vi "OverwriteIni.vi"() -> ()   [LabVIEW 2019]
uses:
  <vilib>/Utility/config.llb/NI_LVConfig.lvlib
  <vilib>/Utility/config.llb/Read Key (String).vi
panel:
  in  "configuration file path":path
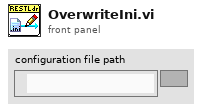
[diagram p1: front panel]
types:
  T1 = typedef "NI_LVConfig.lvlib/Config Data RefNum.ctl" = refnum<k1>
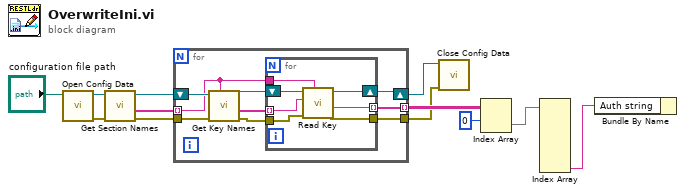
[diagram p0: block diagram]
diagram:
  n1 = call <vilib>:"Open Config Data.vi"("configuration file path"="configuration file path") -> ("error out"=w10:errorcluster, "refnum"=w11:T1)  [unwired: 8 in, 1 out]
  n2 = call <vilib>:"Get Section Names.vi"("error in (no error)"=w10, "refnum"=w11) -> ("error out"=w9:errorcluster, "section names"=w7:string[], "refnum out"=w8:T1)  [unwired: 7 in]
  n3 = for {
    tunnel: w7 -> [w16] mode=indexing
    shift-right: [w18] -> w5
    shift-left: w8 -> [w20]
    tunnel: w9 -> [w21]
    tunnel: [w15] -> w4
    tunnel: [w13] -> w6 mode=indexing
    n4 = call <vilib>:"Get Key Names.vi"("section"=w16, "error in (no error)"=w21, "refnum"=w20) -> ("error out"=w14:errorcluster, "key names"=w17:string[], "refnum out"=w19:T1)  [unwired: 5 in, 1 out]
    n5 = for {
      shift-right: [w27] -> w18
      shift-left: w19 -> [w28]
      tunnel: w17 -> [w26] mode=indexing
      tunnel: w16 -> [w25]
      tunnel: [w24] -> w15
      tunnel: w14 -> [w23]
      tunnel: [w22] -> w13 mode=indexing
      n6 = call-poly <vilib>:"Read Key.vi"("section"=w25, "error in (no error)"=w23, "key"=w26, "refnum"=w28) -> ("error out"=w24:errorcluster, "value"=w22:string, "refnum out"=w27:T1)  [unwired: 4 in, 1 out]
    }
  }
  n7 = call <vilib>:"Close Config Data.vi"("error in (no error)"=w4, "refnum"=w5) -> ()  [unwired: 8 in, 2 out]
  n8 = Index Array(array=w6, index (row)=0) -> (element=w2:string[])  [unwired: 1 in]
  n9 = Index Array(array=w2) -> (element #7=w1:string)  [unwired: 7 in, 6 out]
  n10 = Bundle By Name("Auth string"=w1) -> ()  [unwired: 1 in, 1 out]
